vi "Write_to_OPC.vi"() -> ()   [LabVIEW 2021]
panel:
  in  "Enum":T1(ring)
  in  "stop":bool
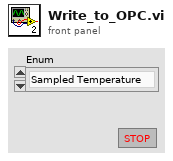
[diagram p1: front panel]
types:
  T1 = enum16{"Sampled Temperature", "Simulated Temperature"}
  T2 = enum16{"Read", "Write", "ReadWrite", "BufferedRead", "BufferedReadWrite"}
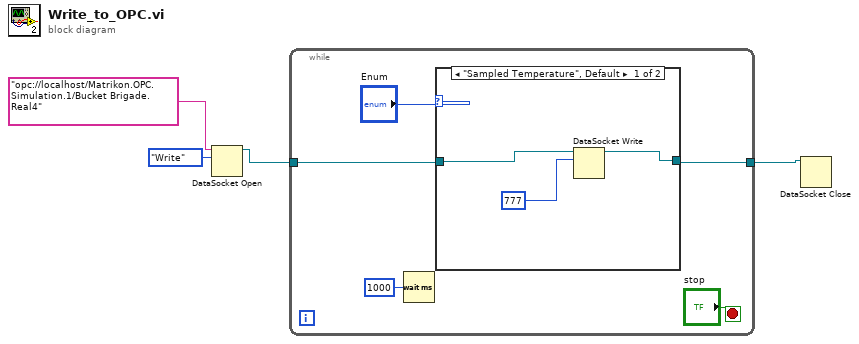
[diagram p0: block diagram]
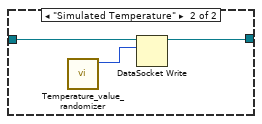
[diagram p2: hidden frame]
diagram:
  n1 = DataSocket Open(10:T2."Write" ("mode"), 11:"opc://localhost/Matrikon.OPC.Simulation.1/Bucket Brigade.Real4") -> (3:w3:refnum<k13>)  [unwired: 2 in, 1 out]
  n2 = while {
    tunnel: w3 -> [w6]
    tunnel: [w5] -> w2
    stop <- "stop" stop-if-true
    n3 = Wait (ms)(milliseconds to wait=u32 1000) -> ()  [unwired: 1 out]
    n4 = case shown="\"Sampled Temperature\", Default" "Enum" {
      tunnel: w6 -> [w12 w15]
      tunnel: [w11 w14] -> w5
      frame "Sampled Temperature", Default {
        n5 = DataSocket Write(10:777, 11:w12) -> (3:w11:refnum<k13>)  [unwired: 2 in, 2 out]
      }
      frame "Simulated Temperature" {
        n6 = call "Temperature_value_randomizer.vi"() -> ("Temperature Value"=w13:i32)  [unwired: 11 in]
        n7 = DataSocket Write(10:w13, 11:w15) -> (3:w14:refnum<k13>)  [unwired: 2 in, 2 out]
      }
    }
  }
  n8 = DataSocket Close(11:w2) -> ()  [unwired: 2 in, 2 out]
